vi "Cheby 2D array prep.vi"   [LabVIEW 2021]
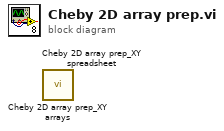
[diagram p0: block diagram]
diagram:
  n1 = call "Cheby 2D array prep_XY arrays.vi"() -> ()  [unwired: 9 in, 2 out]
  n2 = call "Cheby 2D array prep_XY spreadsheet.vi"() -> ()  [unwired: 9 in, 2 out]
